vi "Set AGC Mode.vi"(8 "error in (no error)":errorcluster, 10 "AGC Enable":bool, 11 "RTL-SDR in":refnum<class "RTL-SDR.lvclass">) -> (0 "error out":errorcluster, 1 "function return":i32, 3 "RTL-SDR out":refnum<class "RTL-SDR.lvclass">)   [LabVIEW 2015, in "RTL-SDR.lvclass"]
doc: "Created IvanLis by LabVIEW Portal\nProfile: http://labviewportal.org/memberlist.php?mode=viewprofile&u=987\neMail: IvanLisanov@gMail.com\nTelegram: https://t.me/IvanLis"
uses:
  RTL-SDR.lvclass
  RTL-SDR.lvclass/RTL-SDR.ctl
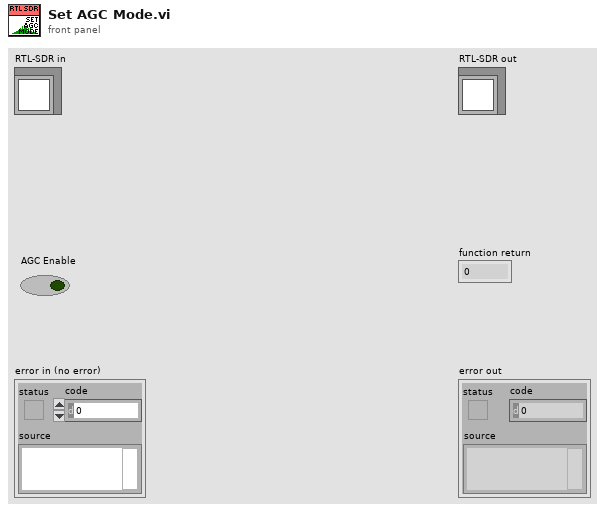
[diagram p1: front panel]
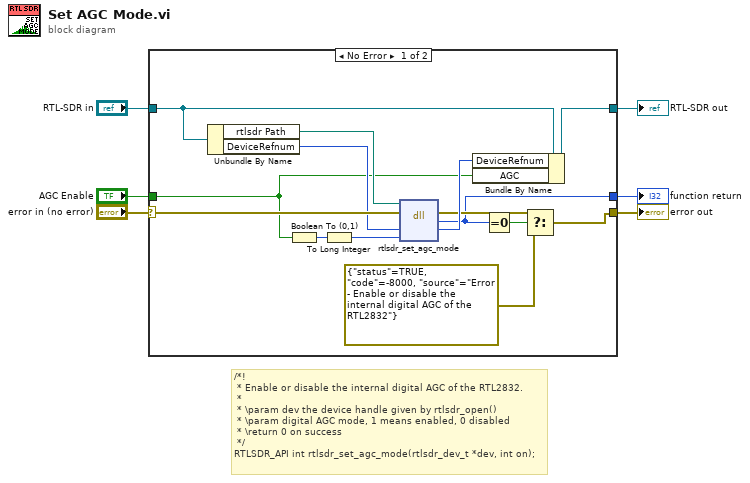
[diagram p0: block diagram]
diagram:
  # "/*!\n * Enable or disable the internal digital AGC of the RTL2832.\n *\n * \\param dev the device handle given by rtlsdr_open()\n * \\param digital AGC mode, 1 means enabled, 0 disabled\n * \\return 0 on success\n */\nRTLSDR_API int rtlsdr_set_agc_mode(rtlsdr_dev_t *dev, int on);"
  n1 = case shown="No Error" "error in (no error)" {
    selector: "error in (no error)" -> [w20 w22]
    tunnel: [w8 w22] -> w5
    tunnel: [w18 w21] -> w3
    tunnel: "RTL-SDR in" -> [w19 w21]
    tunnel: [w7 _] -> w2
    tunnel: "AGC Enable" -> [w12 _]
    frame No Error {
      n2 = Unbundle By Name(w19) -> ("rtlsdr Path"=w16:path, "DeviceRefnum"=w17:u64)
      n3 = Boolean To (0,1)(Boolean=w12) -> (0, 1=w14:i16)
      n4 = To Long Integer(number=w14) -> (32bit integer=w13:i32)
      n5 = dll-call lib="C:/Users/Ivan/Desktop/D-23-09-24 (RTL-SDR)/Project (Pelleng-SDR)/rtlsdr/dll/rtlsdr.*" fn="rtlsdr_set_agc_mode"(path in=w16, error in=w20, "DeviceRefnum"=w17, "AGC Mode"=w13) -> (error out=w9:errorcluster, "return type"=w7:i32, "DeviceRefnum"=w15:u64)  [unwired: 2 in, 1 out]
      n6 = Bundle By Name(cluster=w19, "DeviceRefnum"=w15, "AGC"=w12) -> (w18:refnum<class "RTL-SDR.lvclass">)
      n7 = Equal To 0?(x=w7) -> (x = 0?=w11:bool)
      n8 = Select(t=w9, s=w11, f=errorcluster {"status"=TRUE, "code"=-8000, "source"="Error - Enable or disable the internal digital AGC of the RTL2832"} ("error out")) -> (s? t:f=w8:errorcluster)
    }
    frame Error {
    }
  }
  "error out" <- w5
  "RTL-SDR out" <- w3
  "function return" <- w2
